vi "GetComponentNames.vi"() -> (0 "Component Names":T1)   [LabVIEW 2015]
uses:
  Slit/GSP_SLIT_Global.vi
  Primary Filter/GSP_F1_Global.vi
  Secondary Filter/GSP_F2_Global.vi
  Grating_Translation/GSP_GT_Global.vi
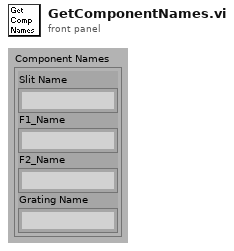
[diagram p1: front panel]
types:
  T1 = cluster{"Slit Name":string, "F1_Name":string, "F2_Name":string, "Grating Name":string}
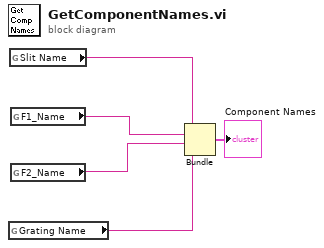
[diagram p0: block diagram]
diagram:
  n1 = global read "GSP_GT_Global.vi" "Grating Name"() -> (w2:string)
  n2 = global read "GSP_SLIT_Global.vi" "Slit Name"() -> (w5:string)
  n3 = global read "GSP_F1_Global.vi" "F1_Name"() -> (w4:string)
  n4 = global read "GSP_F2_Global.vi" "F2_Name"() -> (w3:string)
  n5 = Bundle("Slit Name"=w5, "F1_Name"=w4, "F2_Name"=w3, "Grating Name"=w2) -> (→"Component Names":T1)  [unwired: 1 in]
